vi "C1G2_Assemble CW Only.vi"(7 "Symbol Rate":dbl=10000000.0 format="%#_6p", 11 "Parameters Symbols":T1={"Tari"=8e-06, "PW"=0.5, "factor for \"1\" symbol"=0.5, "RTcal"=2.5, "TRcal"=3.0, "Delimiter"=1.25e-05} {"TRcal" min=1.1 max=3.0 step=0.1; "RTcal" min=2.5 max=3.0 step=0.1; "factor for \"1\" symbol" min=0.5 max=1.0 step=0.1; "PW" min=0.265 max=0.525 step=0.001; "Tari" format="%#_3p"}) -> (2 "Signal out":u8[](array[numeric]))   [LabVIEW 2015]
panel:
  out "Symbols":i32=53374
  out "Digital Waveform":waveform(u8)(graph)={"t0"=timestamp(0 s since 1904-01-01), "dt"=1e-07, "Y"=array[53374 elements]}
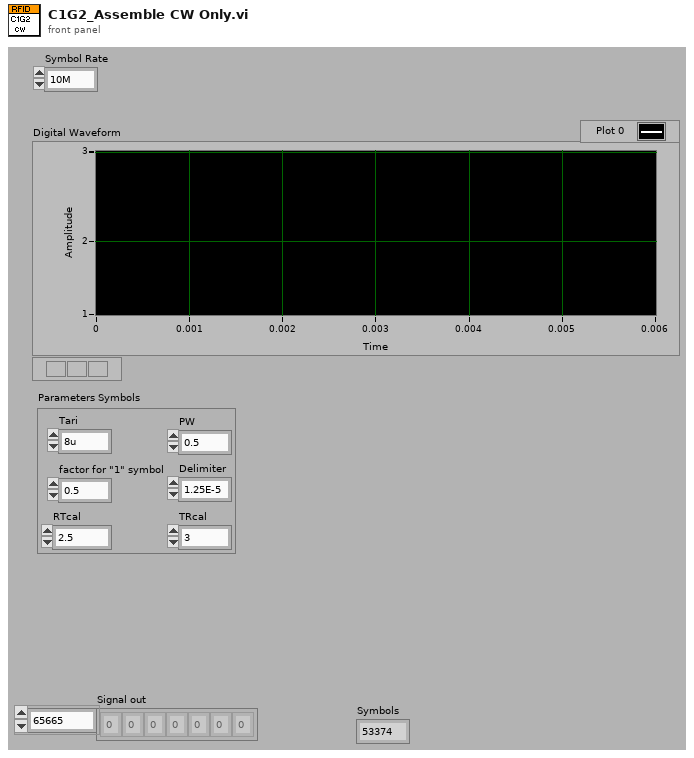
[diagram p1: front panel]
types:
  T1 = cluster{"Tari":dbl, "PW":dbl, "factor for \"1\" symbol":dbl, "RTcal":dbl, "TRcal":dbl, "Delimiter":dbl}
  T2 = typedef "C1G2_BasicsData.ctl" = cluster{"Symbol \"0\"":u8[], "Symbol \"1\"":u8[], "RT Preamble":u8[], "RT Frame Sync":u8[], "Sample Rate":dbl, "LOW-Pulse":u8[], "HIGH-Pulse":u8[], "RT cal":u8[]}
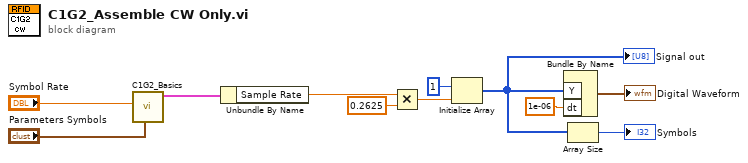
[diagram p0: block diagram]
diagram:
  n1 = call "C1G2_Basics.vi"("Parameters Symbols"="Parameters Symbols", "Symbol Rate"="Symbol Rate") -> ("Basic Components"=w6:T2)  [unwired: 8 in, 1 out]
  n2 = Unbundle By Name(w6) -> ("Sample Rate"=w5:dbl)
  n3 = Multiply(x=w5, y=0.2625 ("Pause length /s")) -> (x*y=w3:dbl)
  n4 = Initialize Array(u8 1 ("element"), w3) -> (w1:u8[])
  "Signal out" <- w1
  n5 = Bundle By Name("Y"=w1, "dt"=1e-06) -> (→"Digital Waveform":waveform(u8))  [unwired: 1 in]
  n6 = Array Size(array=w1) -> (size(s)=→"Symbols":i32)
